vi "Read.vi"(8 "error in (no error)":errorcluster caption="entrée d'erreur (pas d'erreur)", 11 "Class CSV_File (Default) en entrée":refnum<class "Class File (Default).lvclass">) -> (0 "error out":errorcluster caption="sortie d'erreur", 3 "Class CSV_File (Default) en sortie":refnum<class "Class File (Default).lvclass">)   [LabVIEW 2020, in "Library Instrument & Equipement.lvlib" / "Library File.lvlib" / "Class File (Default).lvclass"]
doc: "Reads one or more lines depending on the data condition. If the condition is empty, then the line data is taken into account and the function returns the requested line.\nIf the line value is -1, the entire contents of the file will be returned."
uses:
  Class File (Default).lvclass
  Class File (Default).lvclass/Class File (Default).ctl
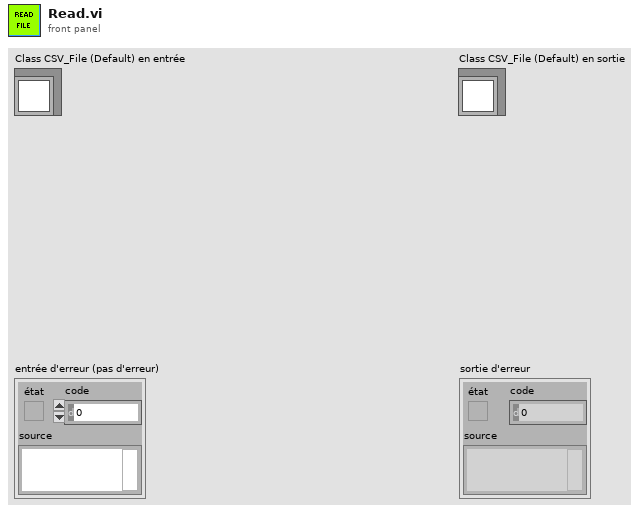
[diagram p1: front panel]
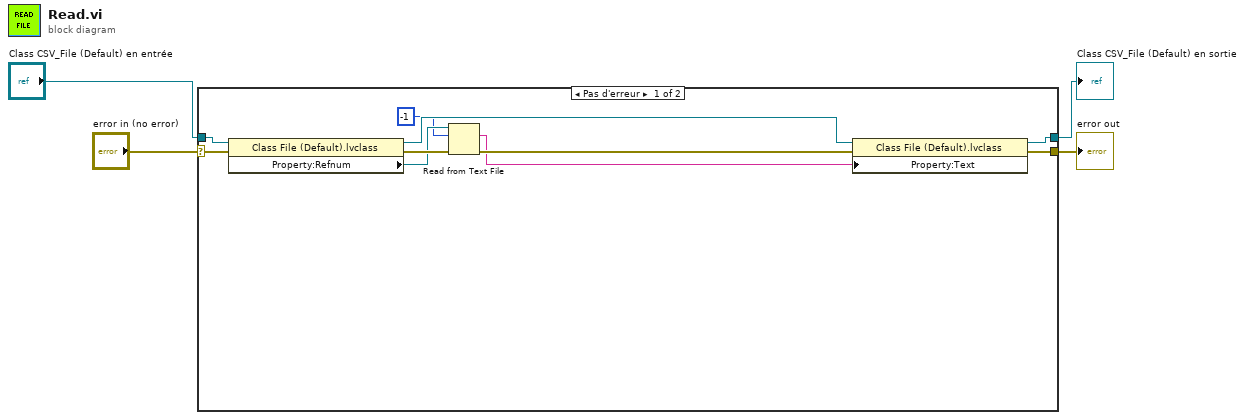
[diagram p0: block diagram]
diagram:
  n1 = case shown="Pas d'erreur" "error in (no error)" {
    selector: "error in (no error)" -> [w13 w16]
    tunnel: [w7 w16] -> w3
    tunnel: [w9 w15] -> w1
    tunnel: "Class CSV_File (Default) en entrée" -> [w14 w15]
    frame No Error {
      n2 = property class="Class File (Default).lvclass"(reference=w14, error in=w13) -> (reference out=w10:refnum<class "Class File (Default).lvclass">, error out=w12:errorcluster, "Property:Refnum"=w11:refnum<file>)
      n3 = Read from Text File(file (use dialog)=w11, count=-1 ("nombre"), error in=w12) -> (text=w5:string, error out=w8:errorcluster)  [unwired: 1 in, 2 out]
      n4 = property class="Class File (Default).lvclass"(reference=w10, error in=w8, "Property:Text"=w5) -> (reference out=w9:refnum<class "Class File (Default).lvclass">, error out=w7:errorcluster)
    }
    frame Error {
    }
  }
  "error out" <- w3
  "Class CSV_File (Default) en sortie" <- w1
